vi "ADSB UI.SetData.vi"(8 "error in (no error)":errorcluster, 10 "Data In":string, 11 "ADSB UI":refnum<class "ADSB UI.lvclass">) -> (0 "error out":errorcluster, 3 "ADSB UI out":refnum<class "ADSB UI.lvclass">)   [LabVIEW 2020, in "ADSB UI.lvclass"]
doc: "---------------------------------------------------------------\nJKI State Machine Objects™\nhttp://jki.net/state-machine-objects/\nCopyright (C) 2005-2015, JKI <info@jki.net>\nALL RIGHTS RESERVEDJKI State Machine Objects (SMO) 1.0.0.5\nJKI - JKI\nCopyright (c) 2016, JKI"
uses:
  ADSB UI.lvclass
  Typedefs/DataChanged--EventData--Cluster.ctl
  ADSB UI.lvclass/ADSB UI.ctl
panel:
  # "For instructions on how to use the JKI State Machine Objects, examples and video tutorials, visit:\nhttp://jki.net/state-machine-objects/\n\nJKI State Machine Objects™\nhttp://jki.net/state-machine-objects/\nCopyright (C) 2005-2015, JKI <info@jki.net>\nALL RIGHTS RESERVED"
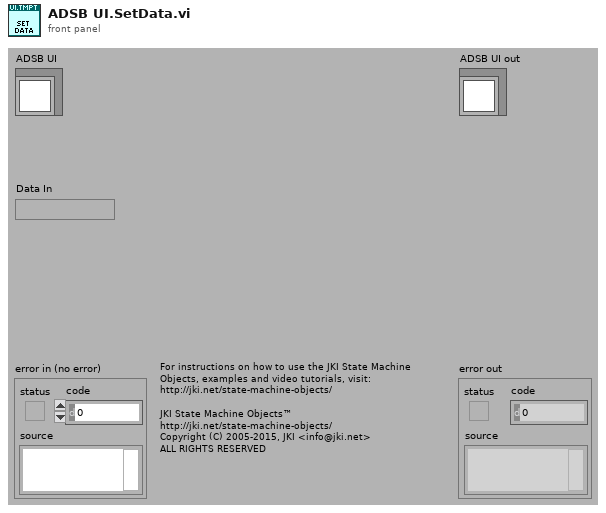
[diagram p1: front panel]
types:
  T1 = typedef "ADSB UI.lvclass/DataChanged--EventData--Cluster.ctl" = cluster{"Timestamp":timestamp, "Old Value":string, "New Value":string}
  T2 = typedef "ADSB UI.lvclass/PrivateData--Ref.ctl" = refnum<data-value>
  T3 = typedef "ADSB UI.lvclass/PrivateData--Cluster.ctl" = cluster{"Configuration":T4, "Public Events":T5, "Protected Events":T6, "Data":string}
  T4 = typedef "ADSB UI.lvclass/Configuration--Cluster.ctl" = cluster{"Suffix":string}
  T5 = typedef "ADSB UI.lvclass/PublicEvents--Cluster.ctl" = cluster{"Data Changed":refnum<user-event>}
  T6 = typedef "ADSB UI.lvclass/ProtectedEvents--Cluster.ctl" = cluster{"API_Template":refnum<user-event>}
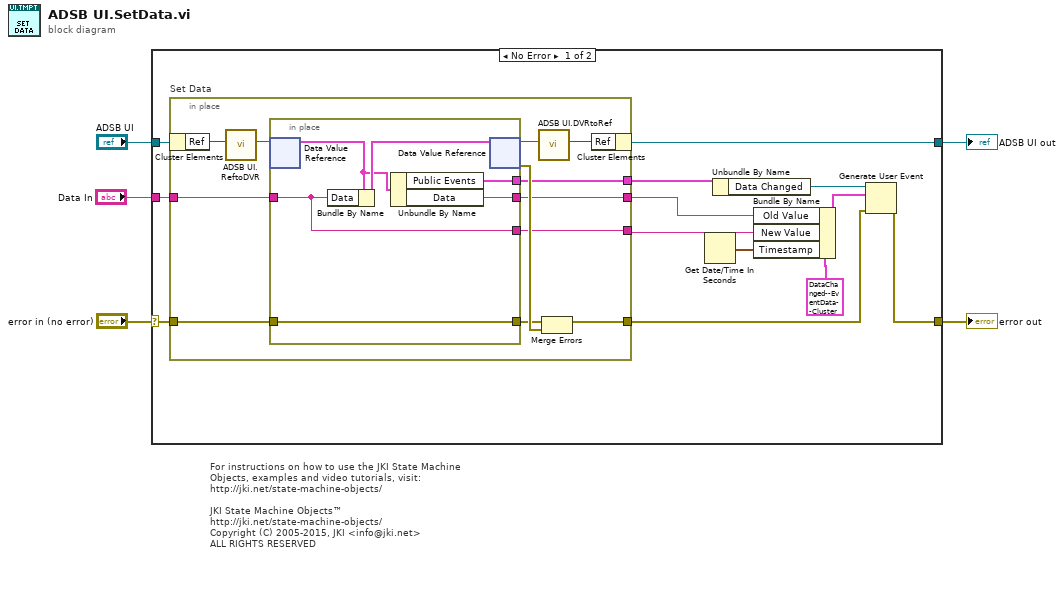
[diagram p0: block diagram]
diagram:
  # "For instructions on how to use the JKI State Machine Objects, examples and video tutorials, visit:\nhttp://jki.net/state-machine-objects/\n\nJKI State Machine Objects™\nhttp://jki.net/state-machine-objects/\nCopyright (C) 2005-2015, JKI <info@jki.net>\nALL RIGHTS RESERVED"
  n1 = case shown="No Error" "error in (no error)" {
    selector: "error in (no error)" -> [w16 w37]
    tunnel: "ADSB UI" -> [w17 w38]
    tunnel: [w7 w37] -> w4
    tunnel: [w15 w38] -> w3
    tunnel: "Data In" -> [w18 _]
    frame No Error {
      n2 = in-place "Set Data" {
        in-place-border: w16 -> [w30]
        in-place-border: [w27] -> w14
        in-place-border: w18 -> [w26]
        in-place-border: [w25] -> w9
        in-place-border: [w24] -> w10
        in-place-border: [w23] -> w6
        n3 = in-place-cluster #1(w17) -> ("Ref"=w22:u32)
        n4 = call "ADSB UI.ReftoDVR.vi"("Ref"=w22) -> ("Ref"=w21:T2)  [unwired: 10 in]
        n5 = in-place {
          in-place-border: w30 -> [w36]
          in-place-border: [w36] -> w28
          in-place-border: w26 -> [w34]
          in-place-border: [w34] -> w25
          in-place-border: [w33] -> w24
          in-place-border: [w31] -> w23
          n6 = in-place-dvr #2(w21) -> (w32:T3)  [unwired: 1 out]
          n7 = Bundle By Name(cluster=w32, "Data"=w34) -> (w35:T3)
          n8 = Unbundle By Name(w32) -> ("Public Events"=w31:T5, "Data"=w33:string)
          n9 = in-place-dvr #2(w35) -> (w20:T2, w29:errorcluster)
        }
        n10 = call "ADSB UI.DVRtoRef.vi"("Ref"=w20) -> ("Ref"=w19:u32)  [unwired: 10 in]
        n11 = Merge Errors(w28, w29) -> (w27:errorcluster)
        n12 = in-place-cluster #1("Ref"=w19) -> (w15:refnum<class "ADSB UI.lvclass">)
      }
      n13 = Get Date/Time In Seconds() -> (seconds since 1Jan1904=w8:timestamp)
      n14 = Unbundle By Name(w6) -> ("Data Changed"=w13:refnum<user-event>)
      n15 = Bundle By Name(cluster=T1 {"Timestamp"=timestamp(0 s since 1904-01-01), "Old Value"="", "New Value"=""} ("event data"), "Old Value"=w10, "New Value"=w9, "Timestamp"=w8) -> (w11:T1)
      n16 = Generate User Event(user event=w13, event data cluster=w11, error in=w14) -> (error out=w7:errorcluster)  [unwired: 1 in, 1 out]
    }
    frame Error {
    }
  }
  "error out" <- w4
  "ADSB UI out" <- w3
